vi "Turn.vi"(10 "Gyro":dbl format="%#_13g", 11 "Effort":dbl) -> ()   [LabVIEW 2016]
uses:
  <vilib>/Rock Robotics/WPI/SafetyOutput/WPI_SafetyOutputConfigMenu.ctl
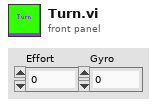
[diagram p1: front panel]
types:
  T1 = typedef "WPI_SafetyOutputConfigMenu.ctl" = enum16{"Enable", "Disable"}
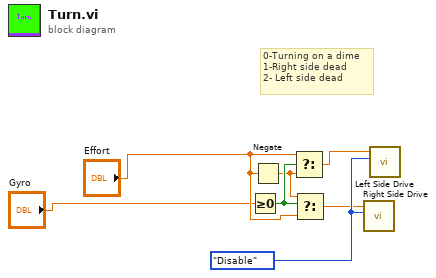
[diagram p0: block diagram]
diagram:
  w7 = WPI_SafetyOutputConfigMenu."Disable" ("mode")
  # "0-Turning on a dime\n1-Right side dead\n2- Left side dead"
  n1 = Greater Or Equal To 0?(x="Gyro") -> (x >= 0?=w6:bool)
  n2 = Negate(x="Effort") -> (-x=w5:dbl)
  n3 = Select(t="Effort", s=w6, f=w5) -> (s? t:f=w1:dbl)
  n4 = Select(t=w5, s=w6, f="Effort") -> (s? t:f=w2:dbl)
  n5 = call "Right Side Drive.vi"("mode"=w7, "Effort"=w2) -> ()  [unwired: 10 in]
  n6 = call "Left Side Drive.vi"("mode"=w7, "Effort"=w1) -> ()  [unwired: 10 in]
